vi "Queue Decorate.vi"(10 "Queue Actor":refnum<class "Queue Actor.lvclass">, 11 "jettl Queue Actor in":refnum<class "jettl Queue Actor.lvclass">) -> (3 "jettl Queue Actor out":refnum<class "jettl Queue Actor.lvclass">)   [LabVIEW 2021, in "jettl Queue Actor.lvlib" / "jettl Queue Actor.lvclass"]
uses:
  jettl Queue Actor.lvclass
  jettl Queue Actor.lvclass/jettl Queue Actor.ctl
  Actor/Queue Actor/Queue Actor.lvclass
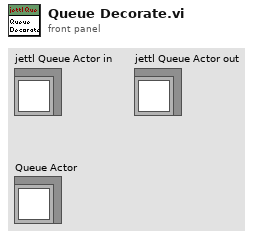
[diagram p1: front panel]
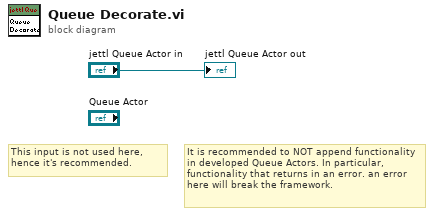
[diagram p0: block diagram]
diagram:
  # "It is recommended to NOT append functionality in developed Queue Actors. In particular, functionality that returns in an error. an error here will break the framework."
  # "This input is not used here, hence it's recommended."
  "jettl Queue Actor out" <- "jettl Queue Actor in"
